vi "zadanie.vi"() -> ()   [LabVIEW 2017]
panel:
  out "Boolean 10":bool
  out "Boolean 12":bool
  out "Boolean 11":bool
  out "Boolean 9":bool
  out "Boolean 8":bool
  in  "stop":bool
  out "Boolean 7":bool
  in  "Boolean 6":bool
  in  "Boolean 5":bool
  in  "Boolean 4":bool
  in  "Boolean 3":bool
  in  "Boolean 2":bool
  in  "Boolean":bool
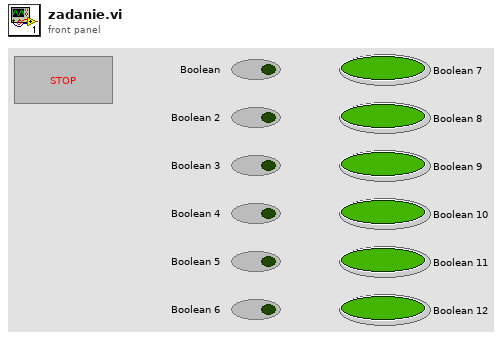
[diagram p1: front panel]
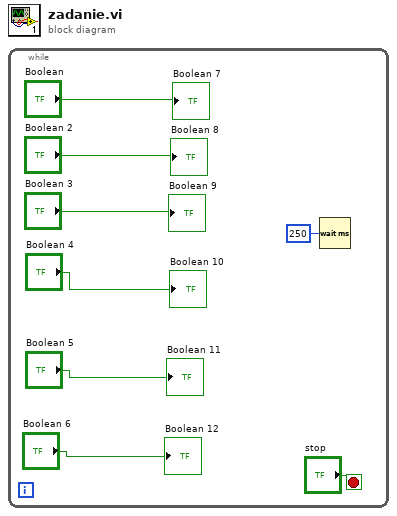
[diagram p0: block diagram]
diagram:
  n1 = while {
    stop <- "stop" stop-if-true
    n2 = Wait (ms)(milliseconds to wait=u32 250) -> ()  [unwired: 1 out]
    "Boolean 7" <- "Boolean"
    "Boolean 8" <- "Boolean 2"
    "Boolean 9" <- "Boolean 3"
    "Boolean 12" <- "Boolean 6"
    "Boolean 11" <- "Boolean 5"
    "Boolean 10" <- "Boolean 4"
  }
